vi "Robot Global Data.vi"() -> ()   [LabVIEW 2016]
doc: "This global VI can contain as many global variables as you need. Place a control on the panel, give it a good name. To read or write to it from a VI, drag the icon to the diagram of that VI. You can also drag from the project. Click on the node to change which global you access. You shouldn't have multiple locations writing to a global or it will cause a race-condition."
uses:
  <vilib>/Rock Robotics/WPI/Camera/WPI_CameraImageSize.ctl
  <vilib>/Rock Robotics/WPI/DriverStation/WPI_DriverStationRobotMode2.ctl
panel:
  in  "Drop Ropes":bool
  in  "Stop Ramping":bool
  in  "Ramp Up Speed":dbl
  in  "Sent Shoot PWM":dbl
  in  "Object Width 2":dbl
  out "Shoot Encoder":dbl
  in  "Voltage Correction Ratio":dbl
  in  "Turning off":bool
  in  "First shoot loop":bool
  in  "Close to peg":bool
  in  "Feeder Speed":dbl=0.9
  in  "Shoot Wheel RPM":dbl
  in  "Run Shoot Wheel":bool
  in  "Ball In Shooter":bool
  in  "Climbing?":bool
  in  "Invert Climb":bool
  in  "Gear Grab Closed":bool
  in  "Gear Up":bool
  in  "Lift Toggle":bool
  in  "Shoot Toggle":bool
  in  "Enable Interval Thump":bool
  in  "Thumper Interval":bool
  in  "NumValuesInTable":dbl
  in  "Gear Grab Release":bool
  in  "Gear Lift Stat":bool
  in  "Gear Box Stat":bool
  in  "Shoot Latch":bool
  in  "Temp Shoot Speed":dbl
  in  "Gear plate pressed?":bool
  in  "Current RPM":dbl=1.0
  in  "Gear In":bool
  in  "Man Gear Latch":bool
  in  "Pixy In Use":bool
  in  "Gear Ready":bool
  in  "Teleop Elapsed":dbl
  in  "Blink":bool
  in  "Warning":bool
  in  "Estop":bool
  in  "RPM 4":dbl=0.85
  in  "RPM 3":dbl=0.95
  in  "RPM 2":dbl=0.9
  in  "RPM 1":dbl=1.0
  in  "RPM Shift":dbl
  in  "Climb Speed":dbl=1.0
  in  "Object Y":dbl
  in  "Gear In Delay":dbl=0.2
  in  "Fast Drive":dbl=100.0
  in  "Slow Drive":dbl=50.0
  in  "Object X":dbl
  in  "Object":bool
  in  "Pixy Output":dbl
  in  "Sonar Distance":dbl
  in  "Robot Mode":T1=enum."Finish"
  in  "image size":T2=enum."320x240"
  in  "Enable Vision":bool
  # "Misc. Variables"
  # "Photon Notification System"
  # "Pixy Vision Processing Variables"
  # "Gear Placement Variables"
  # "Note: Other Variables\nare located in\nPeriodic Tasks"
  # "Passive System"
  # "Used In Periodic"
  # "Shooting Variables"
  # "Note: Other Variables\nare located in\nPeriodic Tasks"
  # "Automated Aiming"
  # "Active System"
  # "Drivetrain Variables"
  # "Climbing"
  # "Unused"
  # "Note: Turn Impementaion\nwas here until a failure\nof another system caused\na rollback. An example is \nin Disabled case of \nDriveControllerBuffer vi"
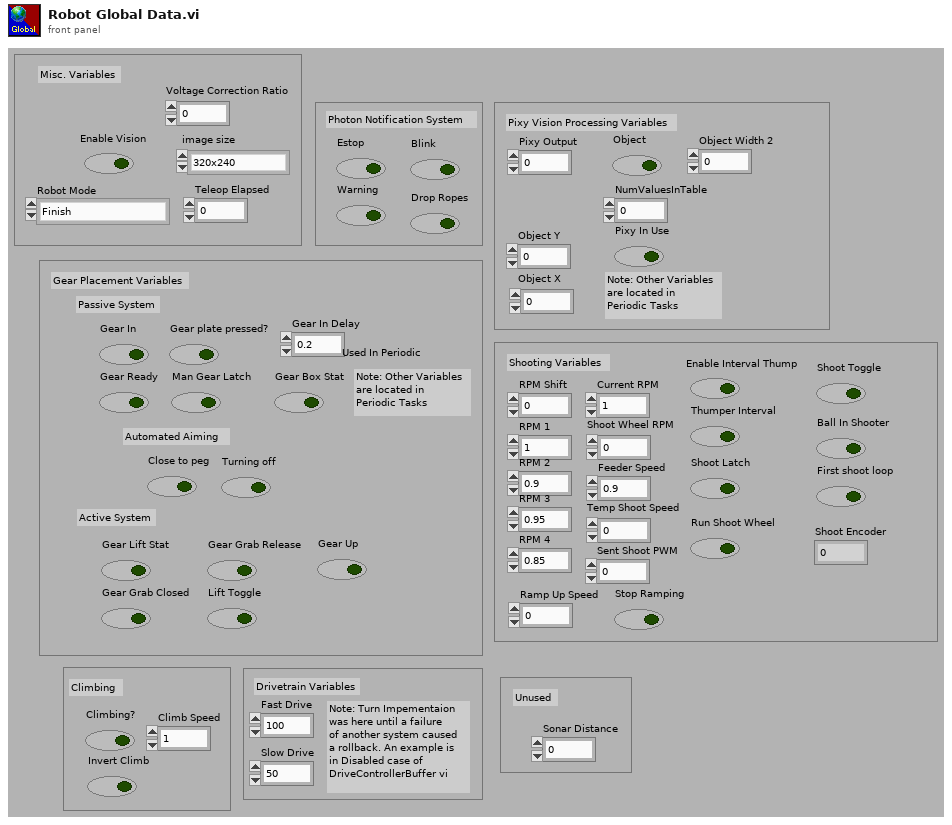
[diagram p1: front panel]
types:
  T1 = typedef "WPI_DriverStationRobotMode2.ctl" = enum16{"Autonomous Disabled", "Autonomous Enabled", "Teleop Disabled", "Teleop Enabled", "Disconnected", "Finish", "Test Disabled", "Test Enabled", "Emergency Stopped"}
  T2 = typedef "WPI_CameraImageSize.ctl" = enum16{"640x480", "320x240", "160x120", "Custom"}
diagram:
